vi "Move To.vi"(8 "error in (no error)":errorcluster, 9 "Index":u16, 10 "Area":enum16{"Home", "Well", "Wash Port"}(ring), 11 "Autosampler in":refnum<class "Autosampler.lvclass">) -> (0 "error out":errorcluster, 3 "Autosampler out":refnum<class "Autosampler.lvclass">)   [LabVIEW 2023, in "Autosampler.lvlib" / "Autosampler.lvclass"]
uses:
  Autosampler.lvclass
  Autosampler.lvclass/Autosampler.ctl
  Autosampler State2.ctl
  Autosampler.lvlib
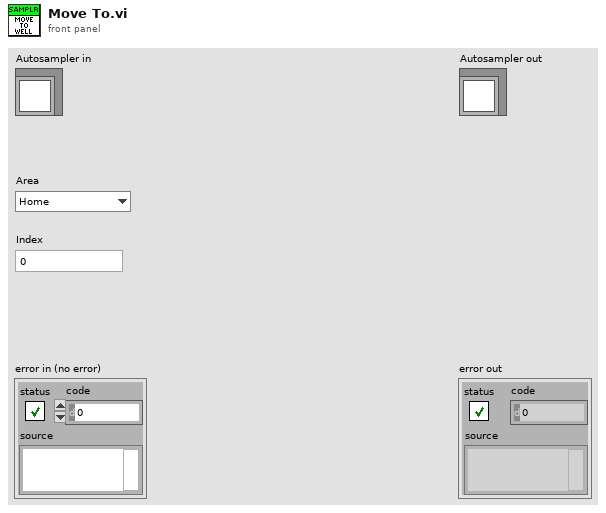
[diagram p1: front panel]
types:
  T1 = typedef "Autosampler.lvlib/Autosampler State2.ctl" = enum16{"Error", "Idle", "Positioning", "Aspirating", "Dispensing", "Washing", "Shaking"}
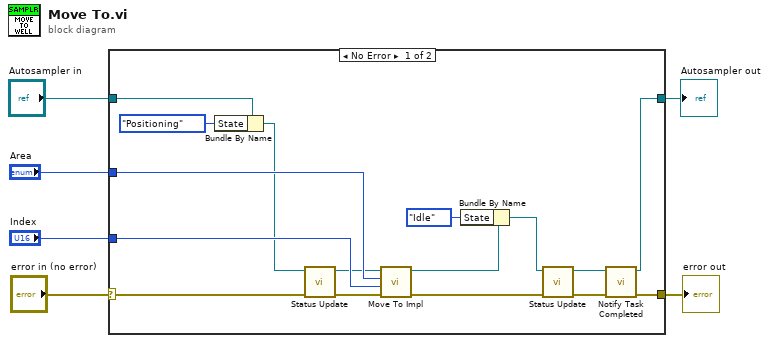
[diagram p0: block diagram]
diagram:
  n1 = case shown="No Error" "error in (no error)" {
    selector: "error in (no error)" -> [w13 w24]
    tunnel: [w17 w24] -> w5
    tunnel: [w16 w23] -> w3
    tunnel: "Autosampler in" -> [w15 w23]
    tunnel: "Area" -> [w22 _]
    tunnel: "Index" -> [w21 _]
    frame No Error {
      n2 = Bundle By Name(cluster=w15, "State"=Autosampler_State2."Positioning") -> (w10:refnum<class "Autosampler.lvclass">)
      n3 = call "Status Update.vi"("error in (no error)"=w13, "Autosampler in"=w10) -> ("error out"=w12:errorcluster, "Autosampler out"=w11:refnum<class "Autosampler.lvclass">)  [unwired: 7 in, 1 out]
      n4 = call-dynamic "Move To Impl.vi"("error in (no error)"=w12, "Index"=w21, "Area"=w22, "Autosampler in"=w11) -> ("error out"=w20:errorcluster, "Autosampler out"=w8:refnum<class "Autosampler.lvclass">)  [unwired: 6 in]
      n5 = Bundle By Name(cluster=w8, "State"=Autosampler_State2."Idle") -> (w7:refnum<class "Autosampler.lvclass">)
      n6 = call "Status Update.vi"("error in (no error)"=w20, "Autosampler in"=w7) -> ("error out"=w19:errorcluster, "Autosampler out"=w18:refnum<class "Autosampler.lvclass">)  [unwired: 7 in, 1 out]
      n7 = call-dynamic "Notify Task Completed.vi"("error in (no error)"=w19, "Device in"=w18) -> ("error out"=w17:errorcluster, "Device out"=w16:refnum<class "Autosampler.lvclass">)  [unwired: 8 in]
    }
    frame Error {
    }
  }
  "error out" <- w5
  "Autosampler out" <- w3
